vi "Front_EndStage.vi"() -> ()   [LabVIEW 2020]
panel:
  out "XY Graph":cluster{"X":dbl, "Y":dbl}[](graph)
  in  "RX Beam Angle":dbl
  in  "RX Beam Angle":dbl
  in  "RX Stage Position":dbl(slide) scale=0.0..10.0
  in  "Beam Gain":dbl
  in  "Beam Angle":dbl
  in  "TX Stage Position":dbl(slide) scale=0.0..10.0
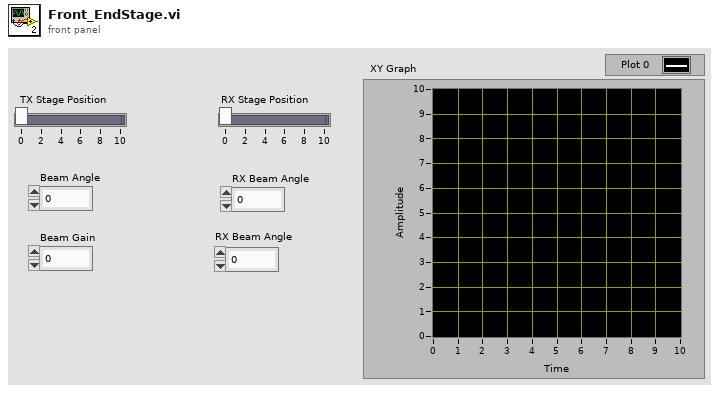
[diagram p1: front panel]
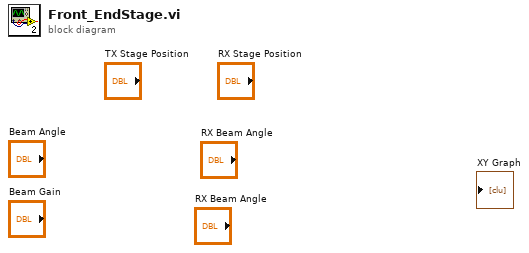
[diagram p0: block diagram]
diagram:
